vi "Get IP Reg Types.vi"(10 "Version":T1, 11 "Engine Simulation IP in":refnum<class "Engine Simulation IP.lvclass">) -> (2 "IP Regs":variant[](array[variant]), 3 "Engine Simulation IP out":refnum<class "Engine Simulation IP.lvclass">)   [LabVIEW 2013, in "Engine Simulation IP.lvclass"]
uses:
  Engine Simulation IP.lvclass
  Bitfile Major Version.ctl
  Engine Simulation Session.lvclass
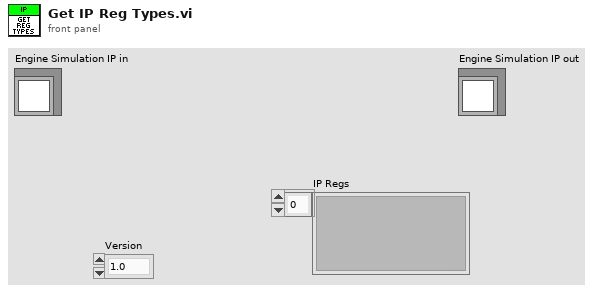
[diagram p1: front panel]
types:
  T1 = typedef "Engine Simulation Session.lvclass/Bitfile Major Version.ctl" = enum16{"1.0", "1.1", "1.2", "1.3"}
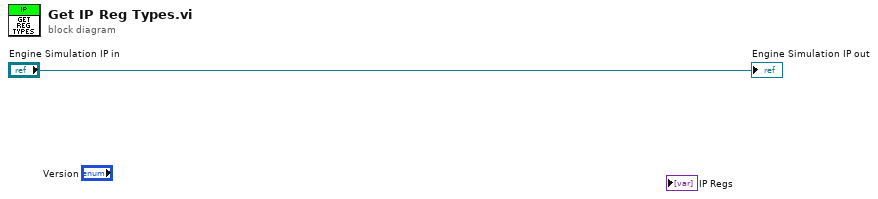
[diagram p0: block diagram]
diagram:
  "Engine Simulation IP out" <- "Engine Simulation IP in"
